vi "ArraysExample_1D.vi"() -> ()   [LabVIEW 2020]
doc: "Example of arrays and related functions. Comments in polish language."
panel:
  in  "Przykładowa tablica":dbl[](array[numeric])
  out "Zbudowana tablica 3":dbl[](array[numeric])
  out "Zbudowana tablica 2":dbl[](array[numeric])
  out "Zbudowana tablica 1":dbl[](array[numeric])
  out "Sinus":dbl[](graph)
  in  "Tablica 9":dbl[](array[numeric])=[4.0, 4.0, 4.0]
  in  "Tablica 8":dbl[](array[numeric])=[3.0, 3.0, 3.0]
  in  "Element 2":dbl=4.0 format="%#_13g"
  in  "Element 1":dbl=4.0 format="%#_13g"
  out "Dodana tablica/element":dbl[](array[numeric])
  in  "Tablica 7":dbl[](array[numeric])=[3.0, 4.0, 5.0, 6.0, 7.0]
  out "Wybrany element":dbl
  in  "Tablica 6":dbl[](array[numeric])=[1.0, 2.0, 3.0, 4.0, 5.0]
  out "Tablica programowa":dbl[](array[numeric])
  out "Rozmiar Tablicy 5":i32
  in  "Tablica 5":dbl[](array[numeric])=[3.0, 2.0, 1.0]
  out "Wynik tablic 2":bool[](array[boolean])
  in  "Tablica 4":bool[](array[boolean])=[FALSE, FALSE, TRUE, FALSE]
  in  "Tablica 3":bool[](array[boolean])=[TRUE, FALSE, FALSE, TRUE]
  out "Wynik tablic 1":dbl[](array[numeric])
  in  "Tablica 2":dbl[](array[numeric])=[11.0, 12.0, 13.0, 14.0]
  in  "Tablica 1":dbl[](array[numeric])=[1.0, 2.0, 3.0, 4.0]
  # "1. Stworzenie najprostszej tablicy liczb i podstawowe parametry tablicy"
  # "2. Działania arymetyczne/logiczne na tablicach"
  # "3. Przegląd funkcji z palety Arrays"
  # "Array size -rozmiar tablicy"
  # "Initialize array-programowe tworzenie tablicy"
  # "Index array-pobranie wartości konkretnego elementu z tablicy"
  # "Insert into array- dodanie elementu bądź innej tablicy"
  # "Build array - budowanie tablic"
  # "4. Pętle i tablice"
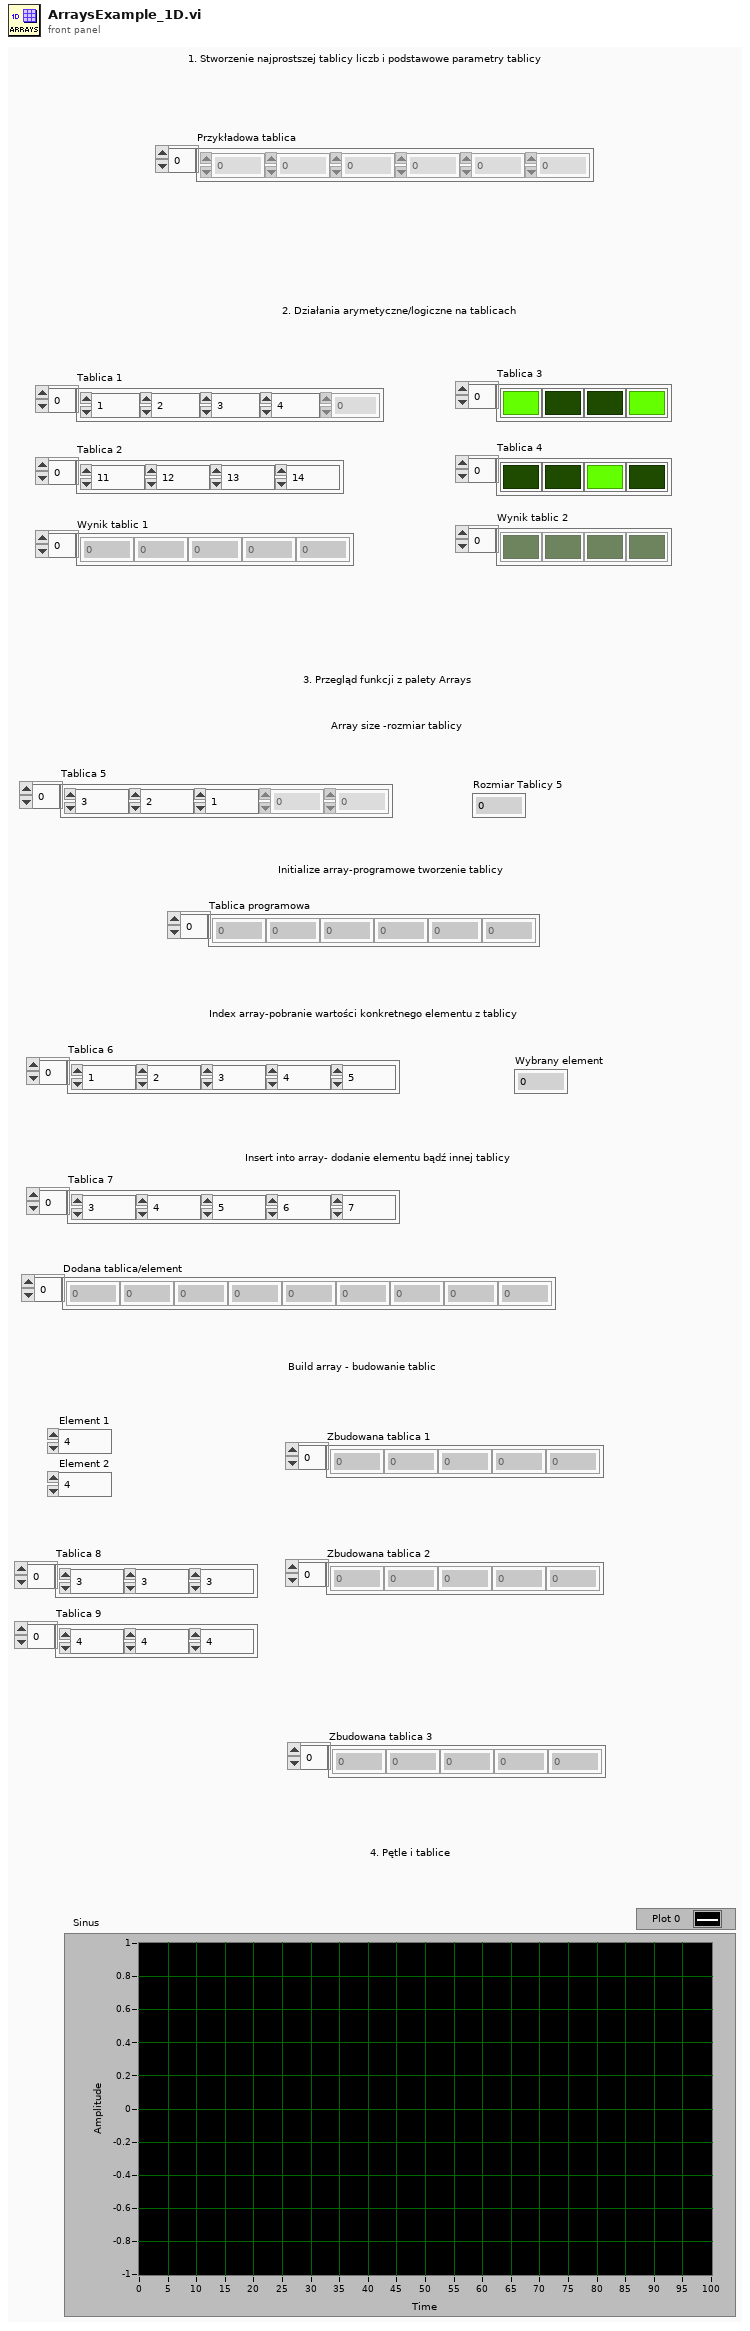
[diagram p1: front panel]
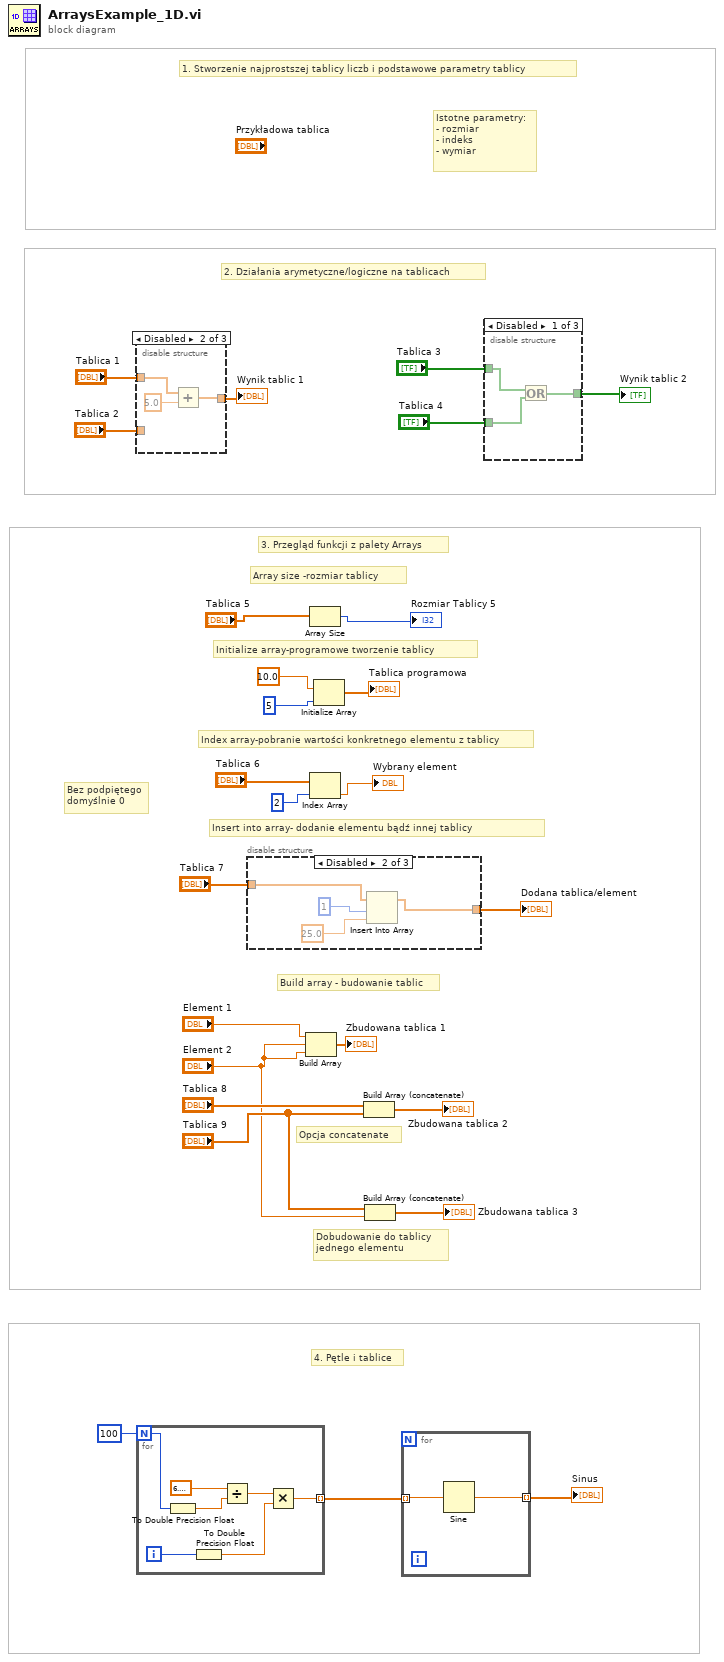
[diagram p0: block diagram]
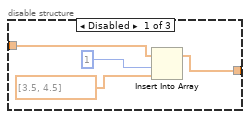
[diagram p2: hidden frame]
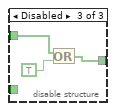
[diagram p5: hidden frame]
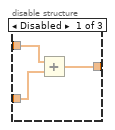
[diagram p6: hidden frame]
diagram:
  # "Bez podpiętego\ndomyślnie 0"
  # "Istotne parametry: \n- rozmiar\n- indeks\n- wymiar"
  # "Dobudowanie do tablicy \njednego elementu"
  # "Opcja concatenate"
  # "4. Pętle i tablice"
  # "Build array - budowanie tablic"
  # "Insert into array- dodanie elementu bądź innej tablicy"
  # "Index array-pobranie wartości konkretnego elementu z tablicy"
  # "Initialize array-programowe tworzenie tablicy"
  # "Array size -rozmiar tablicy"
  # "3. Przegląd funkcji z palety Arrays"
  # "2. Działania arymetyczne/logiczne na tablicach"
  # "1. Stworzenie najprostszej tablicy liczb i podstawowe parametry tablicy"
  n1 = disable-structure shown="Disabled" {
    disable-tunnel: "Tablica 1" -> [w29 w31 _]
    disable-tunnel: "Tablica 2" -> [w28 _ _]
    disable-tunnel: [w27 w30 _] -> w11
    frame Disabled {
      n2 = Add(x=w29, y=w28) -> (x+y=w27:dbl[])
    }
    frame Disabled {
      n3 = Add(x=w31, y=5.0) -> (x+y=w30:dbl[])
    }
    frame Enabled {
    }
  }
  "Wynik tablic 1" <- w11
  n4 = for {
    N: 100 -> [w38]
    tunnel: [w34] -> w20 mode=indexing
    i -> [w33]
    n5 = To Double Precision Float(number=w38) -> (double precision float=w37:dbl)
    n6 = To Double Precision Float(number=w33) -> (double precision float=w35:dbl)
    n7 = Divide(x=6.283185307179586, y=w37) -> (x/y=w36:dbl)
    n8 = Multiply(x=w36, y=w35) -> (x*y=w34:dbl)
  }
  n9 = disable-structure shown="Disabled" {
    disable-tunnel: "Tablica 7" -> [w43 w47 _]
    disable-tunnel: [w40 w44 _] -> w1
    frame Disabled {
      n10 = Insert Into Array(array=w43, index=1, new element=dbl[] [3.5, 4.5]) -> (w40:dbl[])
    }
    frame Disabled {
      n11 = Insert Into Array(array=w47, index=1, new element=25.0 ("new element/subarray")) -> (w44:dbl[])
    }
    frame Enabled {
    }
  }
  "Dodana tablica/element" <- w1
  n12 = Build Array("Element 1", "Element 2", "Element 2") -> (→"Zbudowana tablica 1":dbl[])
  n13 = Array Size(array="Tablica 5") -> (size(s)=→"Rozmiar Tablicy 5":i32)
  n14 = Index Array(array="Tablica 6", index=2) -> (element=→"Wybrany element":dbl)
  n15 = Initialize Array(10.0, 5 ("dimension size")) -> (→"Tablica programowa":dbl[])
  n16 = Build Array (concatenate)("Tablica 8", "Tablica 9") -> (→"Zbudowana tablica 2":dbl[])
  n17 = Build Array (concatenate)("Tablica 9", "Element 2") -> (→"Zbudowana tablica 3":dbl[])
  n18 = for {
    tunnel: w20 -> [w49] mode=indexing
    tunnel: [w48] -> w19 mode=indexing
    n19 = Sine(x=w49) -> (sin(x)=w48:dbl)
  }
  "Sinus" <- w19
  n20 = disable-structure shown="Disabled" {
    disable-tunnel: "Tablica 3" -> [w52 _ w54]
    disable-tunnel: "Tablica 4" -> [w51 _ _]
    disable-tunnel: [w50 _ w53] -> w10
    frame Disabled {
      n21 = Or(x=w52, y=w51) -> (x .or. y?=w50:bool[])
    }
    frame Enabled {
    }
    frame Disabled {
      n22 = Or(x=w54, y=TRUE) -> (x .or. y?=w53:bool[])
    }
  }
  "Wynik tablic 2" <- w10
